vi "To String (Array).vi"(0 "Variant in":variant, 5 "indent":i32, 7 "enable LabVIEW extensions? (T)":bool=TRUE, 9 "pretty print? (T)":bool=TRUE, 11 "error in (no error)":errorcluster) -> (4 "String":string, 15 "error out":errorcluster)   [LabVIEW 2017, in "Variant JSON API.lvlib"]
doc: "Flattens the given JSON data to a string."
uses:
  Variant JSON API.lvlib
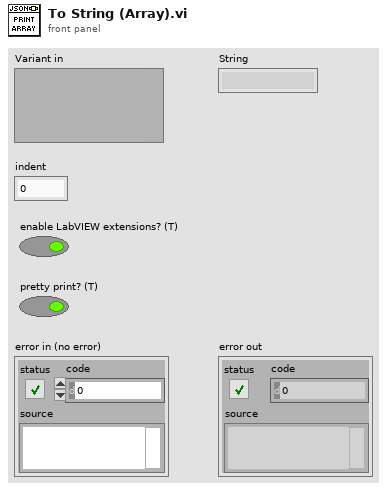
[diagram p1: front panel]
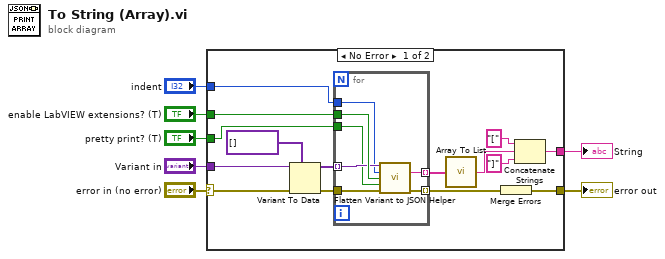
[diagram p0: block diagram]
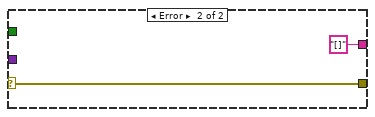
[diagram p2: hidden frame]
diagram:
  n1 = case shown="No Error" "error in (no error)" {
    selector: "error in (no error)" -> [w12 w31]
    tunnel: "Variant in" -> [w14 _]
    tunnel: [w20 w31] -> w5
    tunnel: [w19 "[]"] -> w4
    tunnel: "enable LabVIEW extensions? (T)" -> [w15 _]
    tunnel: "pretty print? (T)" -> [w10 _]
    tunnel: "indent" -> [w9 _]
    frame No Error {
      n2 = Variant To Data(error in=w12, type=variant[] [], Variant=w14) -> (data=w13:variant[], error out=w11:errorcluster)
      n3 = for {
        tunnel: [w23] -> w22 mode=indexing
        tunnel: w11 -> [w29]
        tunnel: [w28] -> w21 mode=indexing
        tunnel: w15 -> [w27]
        tunnel: w13 -> [w26] mode=indexing
        tunnel: w10 -> [w25]
        tunnel: w9 -> [w24]
        n4 = call "Flatten Variant to JSON Helper.vi"("Variant in"=w26, "indent"=w24, "enable LabVIEW extensions? (T)"=w27, "pretty print? (T)"=w25, "error in (no error)"=w29) -> ("String"=w23:string, "error out"=w28:errorcluster)  [unwired: 8 in, 1 out]
      }
      n5 = call "Array To List.vi"("Array"=w22) -> ("String"=w18:string)  [unwired: 14 in]
      n6 = Merge Errors(w21) -> (w20:errorcluster)
      n7 = Concatenate Strings("[" ("string"), w18, "]" ("string")) -> (w19:string)
    }
    frame Error {
    }
  }
  "String" <- w4
  "error out" <- w5
